vi "Configure Basic Network Connection.vi"(4 "DHCP (Enabled)":bool=TRUE, 5 "NameServer2 (0.0.0.0)":string="0.0.0.0", 6 "Net Mask (255.255.255.0)":string="255.255.255.0", 7 "NameServer1 (192.168.0.1)":string="192.168.0.1", 8 "error in (no error)":errorcluster, 9 "Gateway Address (192.168.0.1)":string="192.168.0.1", 10 "IP Address (192.168.0.112)":string="192.168.0.112", 11 "VISA resource name":refnum<visa-resource-name>) -> (0 "error out":errorcluster, 3 "VISA resource name out":refnum<visa-resource-name>)   [LabVIEW 2013, in "Watts Up Series.lvlib"]
doc: "Basic network configuration for the Watts Up .Net device. Enter your network information in the controls.\n\n<b>Note:</b> The Watts Up .Net will by default find and set these parameters to the device when you connect it to an ethernet port. But if you need to configure them manually then use this VI."
uses:
  <instrlib>/Watts Up Series/Watts Up Series.lvlib
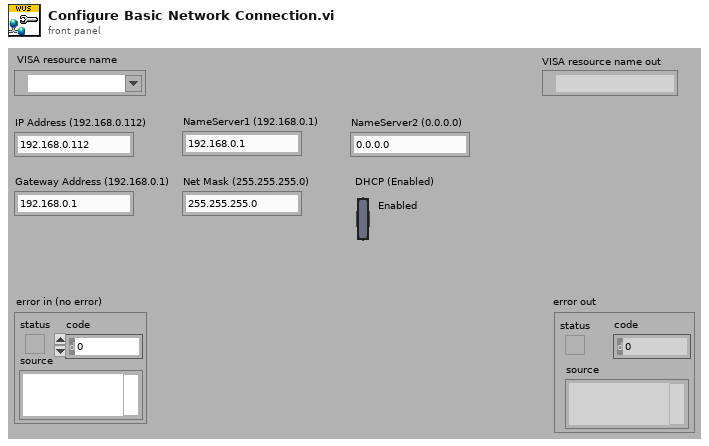
[diagram p1: front panel]
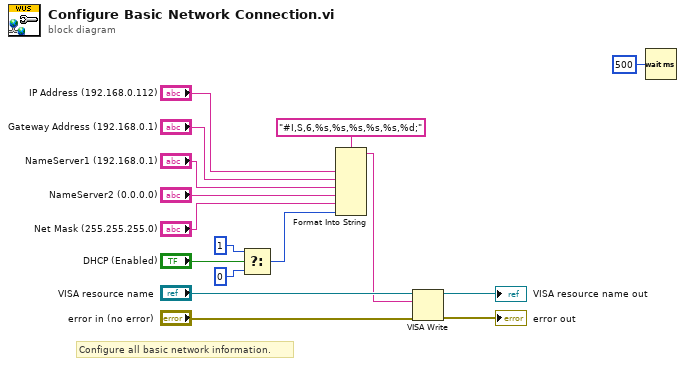
[diagram p0: block diagram]
diagram:
  # "Configure all basic network information."
  n1 = Select(t=1, s="DHCP (Enabled)", f=0) -> (s? t:f=w7:i32)
  n2 = Format Into String(format string="#I,S,6,%s,%s,%s,%s,%s,%d;", "IP Address (192.168.0.112)", "Gateway Address (192.168.0.1)", "NameServer1 (192.168.0.1)", "NameServer2 (0.0.0.0)", "Net Mask (255.255.255.0)", w7) -> (resulting string=w2:string)  [unwired: 2 in, 1 out]
  n3 = VISA Write(VISA resource name="VISA resource name", write buffer=w2, error in (no error)="error in (no error)") -> (VISA resource name out=→"VISA resource name out":refnum<visa-resource-name>, error out=→"error out":errorcluster)  [unwired: 1 out]
  n4 = Wait (ms)(milliseconds to wait=u32 500) -> ()  [unwired: 1 out]
